vi "A-Star Main.vi"() -> ()   [LabVIEW 2009]
panel:
  out "XY Graph 3":cluster{dbl[], dbl[]}[](graph)
  out "XY Graph 2":cluster{"X":dbl, "Y":dbl}[](graph)
  out "XY Graph":cluster{"X":dbl, "Y":dbl}[](graph)
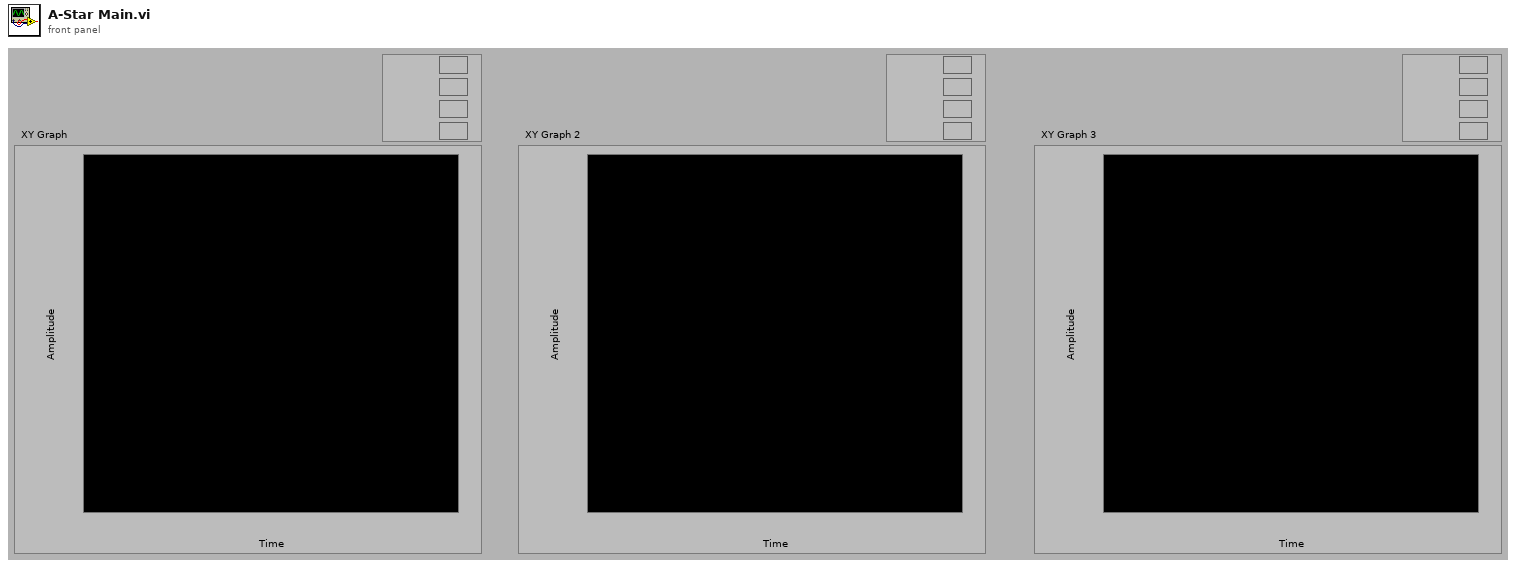
[diagram p1: front panel]
types:
  T1 = cluster{"Square":cluster{"X":dbl, "Y":dbl}, "Parent Square":cluster{"X":dbl, "Y":dbl}, "G":dbl, "H":dbl}[]
  T2 = cluster{"Square":cluster{"X":dbl, "Y":dbl}, "Parent Square":cluster{"X":dbl, "Y":dbl}, "G":dbl, "H":dbl}
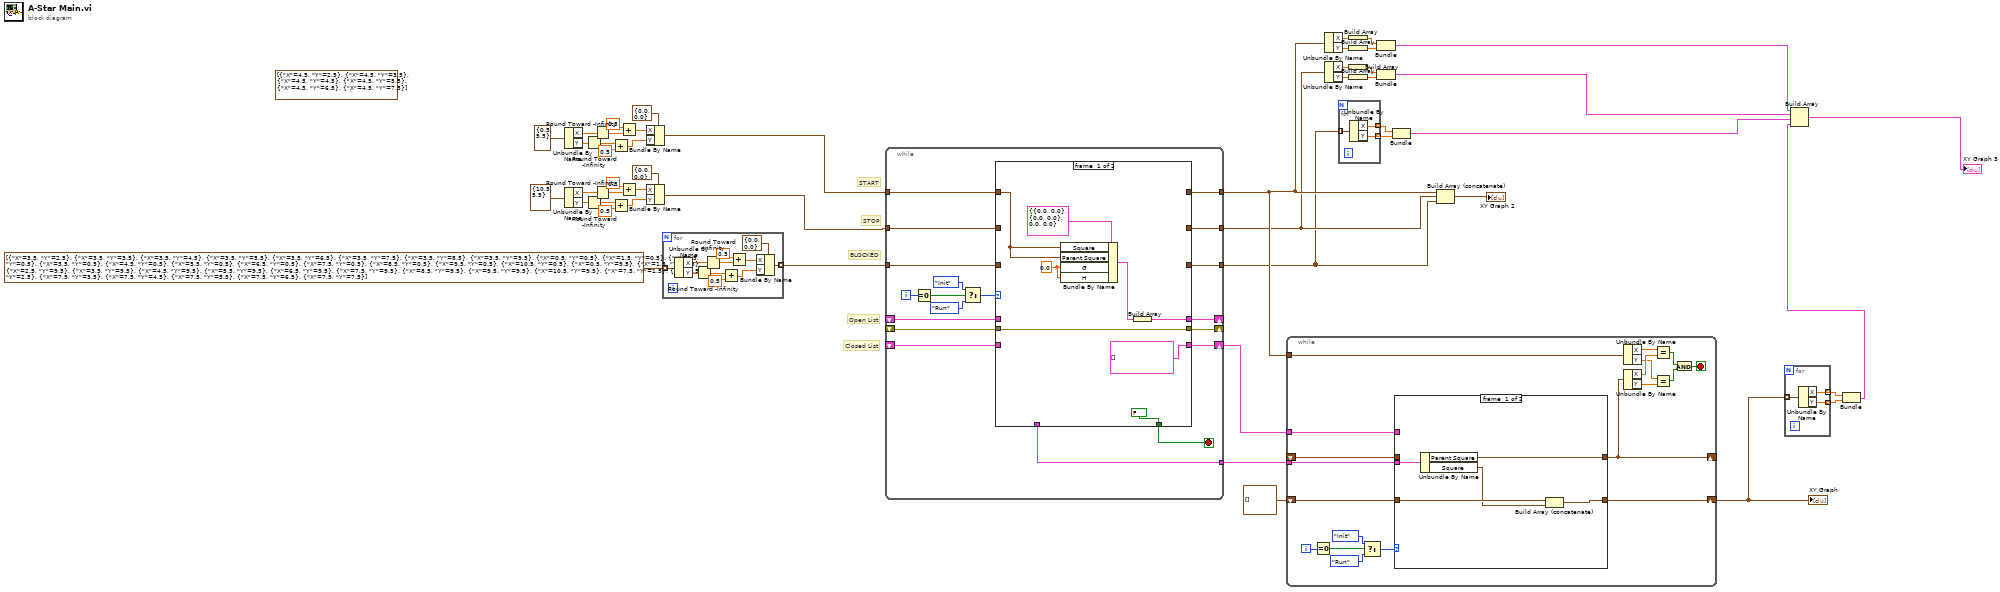
[diagram p0: block diagram]
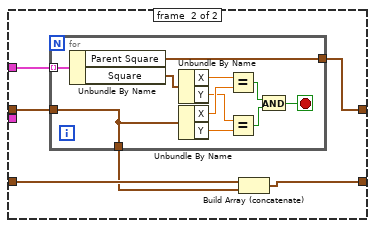
[diagram p2: hidden frame]
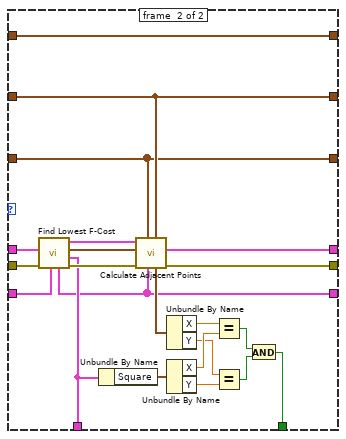
[diagram p3: hidden frame]
diagram:
  (unwired) cluster{"X":dbl, "Y":dbl}[] [{"X"=4.5, "Y"=2.5}, {"X"=4.5, "Y"=3.5}, {"X"=4.5, "Y"=4.5}, {"X"=4.5, "Y"=5.5}, {"X"=4.5, "Y"=6.5}, {"X"=4.5, "Y"=7.5}]
  # "Closed List"
  # "Open List"
  # "BLOCKED"
  # "STOP"
  # "START"
  n1 = Unbundle By Name(cluster{"X":dbl, "Y":dbl} {"X"=0.5, "Y"=5.5} ("Cluster")) -> ("X"=w15:dbl, "Y"=w16:dbl)
  n2 = Unbundle By Name(cluster{"X":dbl, "Y":dbl} {"X"=10.5, "Y"=5.5} ("Cluster")) -> ("X"=w13:dbl, "Y"=w12:dbl)
  n3 = Round Toward -Infinity(1:w16) -> (0:w18:dbl)
  n4 = Round Toward -Infinity(1:w12) -> (0:w10:dbl)
  n5 = Round Toward -Infinity(1:w15) -> (0:w19:dbl)
  n6 = Round Toward -Infinity(1:w13) -> (0:w9:dbl)
  n7 = Add(x=w18, y=0.5) -> (x+y=w23:dbl)
  n8 = Add(x=w10, y=0.5) -> (x+y=w5:dbl)
  n9 = Add(x=0.5, y=w19) -> (x+y=w22:dbl)
  n10 = Add(x=0.5, y=w9) -> (x+y=w6:dbl)
  n11 = Bundle By Name(cluster=cluster{"X":dbl, "Y":dbl} {"X"=0.0, "Y"=0.0} ("Cluster"), "X"=w22, "Y"=w23) -> (w1:cluster{"X":dbl, "Y":dbl})
  n12 = Bundle By Name(cluster=cluster{"X":dbl, "Y":dbl} {"X"=0.0, "Y"=0.0} ("Cluster"), "X"=w6, "Y"=w5) -> (w2:cluster{"X":dbl, "Y":dbl})
  n13 = for {
    tunnel: cluster{"X":dbl, "Y":dbl}[] [{"X"=3.5, "Y"=2.5}, {"X"=3.5, "Y"=3.5}, {"X"=3.5, "Y"=4.5}, {"X"=3.5, "Y"=5.5}, {"X"=3.5, "Y"=6.5}, {"X"=3.5, "Y"=7.5}, {"X"=3.5, "Y"=8.5}, {"X"=3.5, "Y"=9.5}, {"X"=0.5, "Y"=0.5}, {"X"=1.5, "Y"=0.5}, {"X"=2.5, "Y"=0.5}, {"X"=3.5, "Y"=0.5}, {"X"=4.5, "Y"=0.5}, {"X"=5.5, "Y"=0.5}, {"X"=6.5, "Y"=0.5}, {"X"=7.5, "Y"=0.5}, {"X"=8.5, "Y"=0.5}, {"X"=9.5, "Y"=0.5}, {"X"=10.5, "Y"=0.5}, {"X"=0.5, "Y"=9.5}, {"X"=1.5, "Y"=9.5}, {"X"=2.5, "Y"=9.5}, {"X"=3.5, "Y"=9.5}, {"X"=4.5, "Y"=9.5}, {"X"=5.5, "Y"=9.5}, {"X"=6.5, "Y"=9.5}, {"X"=7.5, "Y"=9.5}, {"X"=8.5, "Y"=9.5}, {"X"=9.5, "Y"=9.5}, {"X"=10.5, "Y"=9.5}, {"X"=7.5, "Y"=1.5}, {"X"=7.5, "Y"=2.5}, {"X"=7.5, "Y"=3.5}, {"X"=7.5, "Y"=4.5}, {"X"=7.5, "Y"=5.5}, {"X"=7.5, "Y"=6.5}, {"X"=7.5, "Y"=7.5}] -> [w60] mode=indexing
    tunnel: [w50] -> w3 mode=indexing
    n14 = Unbundle By Name(w60) -> ("X"=w59:dbl, "Y"=w58:dbl)
    n15 = Round Toward -Infinity(1:w58) -> (0:w56:dbl)
    n16 = Round Toward -Infinity(1:w59) -> (0:w55:dbl)
    n17 = Add(x=w56, y=0.5) -> (x+y=w51:dbl)
    n18 = Add(x=0.5, y=w55) -> (x+y=w52:dbl)
    n19 = Bundle By Name(cluster=cluster{"X":dbl, "Y":dbl} {"X"=0.0, "Y"=0.0} ("Cluster"), "X"=w52, "Y"=w51) -> (w50:cluster{"X":dbl, "Y":dbl})
  }
  n20 = while {
    shift-right: [w76] -> _
    shift-left: _ -> [w75]
    tunnel: w3 -> [w77]
    tunnel: w2 -> [w78]
    tunnel: w1 -> [w79]
    shift-right: [w69] -> _
    shift-left: _ -> [w68]
    tunnel: [w66] -> w49
    tunnel: [w65] -> w42
    shift-right: [w64] -> w48
    shift-left: _ -> [w63]
    tunnel: [w62] -> w33
    tunnel: [w61] -> w32
    i -> [w71]
    stop <- w67 stop-if-true
    n21 = Equal To 0?(x=w71) -> (x = 0?=w70:bool)
    n22 = Select(t=enum16{"Init", "Run"}."Init", s=w70, f=enum16{"Init", "Run"}."Run") -> (s? t:f=w72:enum16{"Init", "Run"})
    n23 = case shown="\"Run\"" w72 {
      tunnel: w79 -> [w81 w95]
      tunnel: w78 -> [_ w90]
      tunnel: w77 -> [_ w89]
      tunnel: [w87 w107] -> w76
      tunnel: w75 -> [_ w109]
      tunnel: [w83 w106] -> w69
      tunnel: w68 -> [w83 w105]
      tunnel: [FALSE w96] -> w67
      tunnel: [_ w93] -> w66
      tunnel: [_ w95] -> w65
      tunnel: [T1 [] ("Closed List In") w88] -> w64
      tunnel: w63 -> [_ w94]
      tunnel: [_ w90] -> w62
      tunnel: [_ w89] -> w61
      frame #0 {
        w84 = 0.0 ("G")
        n24 = Bundle By Name(cluster=T2 {"Square"={"X"=0.0, "Y"=0.0}, "Parent Square"={"X"=0.0, "Y"=0.0}, "G"=0.0, "H"=0.0} ("Cluster"), "Square"=w81, "Parent Square"=w81, "G"=w84, "H"=w84) -> (w86:T2)
        n25 = Build Array(w86) -> (w87:T1)
      }
      frame #1 {
        n26 = call "Find Lowest F-Cost.vi"("Closed List In"=w94, "error in (no error)"=w105, "Open List"=w109) -> ("error out"=w108:errorcluster, "Square with Parent"=w93:T2, "Square"=w91:cluster{"X":dbl, "Y":dbl}, "Open List Out"=w92:T1, "Closed List Out"=w88:T1)  [unwired: 4 in]
        n27 = Unbundle By Name(w93) -> ("Square"=w104:cluster{"X":dbl, "Y":dbl})
        n28 = call "Calculate Adjacent Points.vi"("End Point"=w90, "Closed List In"=w88, "Blocked Points"=w89, "error in (no error)"=w108, "Open Point"=w91, "Open List In"=w92) -> ("error out"=w106:errorcluster, "Open List Out"=w107:T1, "End Point Out"=w103:cluster{"X":dbl, "Y":dbl})  [unwired: 3 in]
        n29 = Unbundle By Name(w103) -> ("X"=w102:dbl, "Y"=w99:dbl)
        n30 = Unbundle By Name(w104) -> ("X"=w101:dbl, "Y"=w100:dbl)
        n31 = Equal?(x=w102, y=w101) -> (x = y?=w98:bool)
        n32 = Equal?(x=w99, y=w100) -> (x = y?=w97:bool)
        n33 = And(x=w98, y=w97) -> (x .and. y?=w96:bool)
      }
    }
  }
  n34 = while {
    tunnel: w42 -> [w128]
    tunnel: w49 -> [w115]
    tunnel: w48 -> [w112]
    shift-right: [w113] -> w45
    shift-left: cluster{"X":dbl, "Y":dbl}[] [] -> [w114]
    shift-right: [w110] -> _
    shift-left: _ -> [w111]
    i -> [w117]
    stop <- w121 stop-if-true
    n35 = Equal To 0?(x=w117) -> (x = 0?=w118:bool)
    n36 = Select(t=enum16{"Init", "Run"}."Init", s=w118, f=enum16{"Init", "Run"}."Run") -> (s? t:f=w116:enum16{"Init", "Run"})
    n37 = case shown="\"Run\"" w116 {
      tunnel: w115 -> [w133 _]
      tunnel: w114 -> [w132 w137]
      tunnel: [w130 w135] -> w113
      tunnel: w112 -> [_ w139]
      tunnel: [w129 w134] -> w110
      tunnel: w111 -> [_ w138]
      frame #0 {
        n38 = Unbundle By Name(w133) -> ("Parent Square"=w129:cluster{"X":dbl, "Y":dbl}, "Square"=w131:cluster{"X":dbl, "Y":dbl})
        n39 = Build Array (concatenate)(w132, w131) -> (w130:cluster{"X":dbl, "Y":dbl}[])
      }
      frame #1 {
        n40 = for {
          tunnel: w139 -> [w150] mode=indexing
          tunnel: w138 -> [w141]
          tunnel: [w141] -> w136
          tunnel: [w140] -> w134
          stop <- w142 stop-if-true
          n41 = Unbundle By Name(w150) -> ("Parent Square"=w140:cluster{"X":dbl, "Y":dbl}, "Square"=w149:cluster{"X":dbl, "Y":dbl})
          n42 = Unbundle By Name(w149) -> ("X"=w148:dbl, "Y"=w145:dbl)
          n43 = Unbundle By Name(w141) -> ("X"=w146:dbl, "Y"=w147:dbl)
          n44 = Equal?(x=w148, y=w146) -> (x = y?=w144:bool)
          n45 = Equal?(x=w145, y=w147) -> (x = y?=w143:bool)
          n46 = And(x=w144, y=w143) -> (x .and. y?=w142:bool)
        }
        n47 = Build Array (concatenate)(w137, w136) -> (w135:cluster{"X":dbl, "Y":dbl}[])
      }
    }
    n48 = Unbundle By Name(w128) -> ("X"=w125:dbl, "Y"=w122:dbl)
    n49 = Unbundle By Name(w110) -> ("X"=w123:dbl, "Y"=w124:dbl)
    n50 = Equal?(x=w125, y=w123) -> (x = y?=w126:bool)
    n51 = Equal?(x=w122, y=w124) -> (x = y?=w127:bool)
    n52 = And(x=w126, y=w127) -> (x .and. y?=w121:bool)
  }
  "XY Graph" <- w45
  n53 = Unbundle By Name(w42) -> ("X"=w41:dbl, "Y"=w40:dbl)
  n54 = Unbundle By Name(w33) -> ("X"=w34:dbl, "Y"=w35:dbl)
  n55 = for {
    tunnel: w32 -> [w153] mode=indexing
    tunnel: [w152] -> w30 mode=indexing
    tunnel: [w151] -> w31 mode=indexing
    n56 = Unbundle By Name(w153) -> ("X"=w152:dbl, "Y"=w151:dbl)
  }
  n57 = Build Array(w41) -> (w39:dbl[])
  n58 = Build Array(w40) -> (w38:dbl[])
  n59 = Build Array(w34) -> (w36:dbl[])
  n60 = Build Array(w35) -> (w37:dbl[])
  n61 = Bundle(w39, w38) -> (w29:cluster{dbl[], dbl[]})  [unwired: 1 in]
  n62 = Bundle(w36, w37) -> (w28:cluster{dbl[], dbl[]})  [unwired: 1 in]
  n63 = Bundle(w30, w31) -> (w27:cluster{dbl[], dbl[]})  [unwired: 1 in]
  n64 = Build Array (concatenate)(w42, w33, w32) -> (→"XY Graph 2":cluster{"X":dbl, "Y":dbl}[])
  n65 = for {
    tunnel: w45 -> [w156] mode=indexing
    tunnel: [w155] -> w44 mode=indexing
    tunnel: [w154] -> w43 mode=indexing
    n66 = Unbundle By Name(w156) -> ("X"=w155:dbl, "Y"=w154:dbl)
  }
  n67 = Bundle(w44, w43) -> (w26:cluster{dbl[], dbl[]})  [unwired: 1 in]
  n68 = Build Array(w29, w28, w27, w26) -> (→"XY Graph 3":cluster{dbl[], dbl[]}[])
